vi "paint.vi"() -> ()   [LabVIEW 2017]
uses:
  <vilib>/Utility/inputDevices.llb/mouseAcquire.vi
panel:
  out "Speed":i64
  in  "Speed":T1(radio)
  out "Stop Indicator":bool
  out "Reset Frame":bool
  in  "Stop":bool
  in  "Load 4":bool
  in  "Delete Image 4":bool
  in  "Load 3":bool
  in  "Delete Image 3":bool
  in  "Load 2":bool
  in  "Delete Image 2":bool
  in  "Load 1":bool
  in  "Delete Image 1":bool
  in  "Clear":bool
  out "Saved Images":T2(array[cluster])
  in  "Save":bool
  in  "Delete Line":bool
  in  "Lines":i32(listbox)
  out "Current Image":cluster{"X":i32, "Y":i32}[][](array[cluster])
  out "2D Picture":picture
  # "Click and drag the left mouse button\ninside the black box to draw."
  # "Click on a line in\nthe list to select it.\nUse the Delete Line\nbutton to delete it.\nDeleting with no\nselection clears the\nfirst line in the list."
  # "Click the Save Image and\nClear Image buttons to save or\nclear the current image"
  # "Click STOP to stop the program"
  # "Click the Load Image or Delete Image\nbuttons below one of the saved images\nto load/delete it. Use the scrollbar to\nscroll through saved images."
  # "Laser Speed"
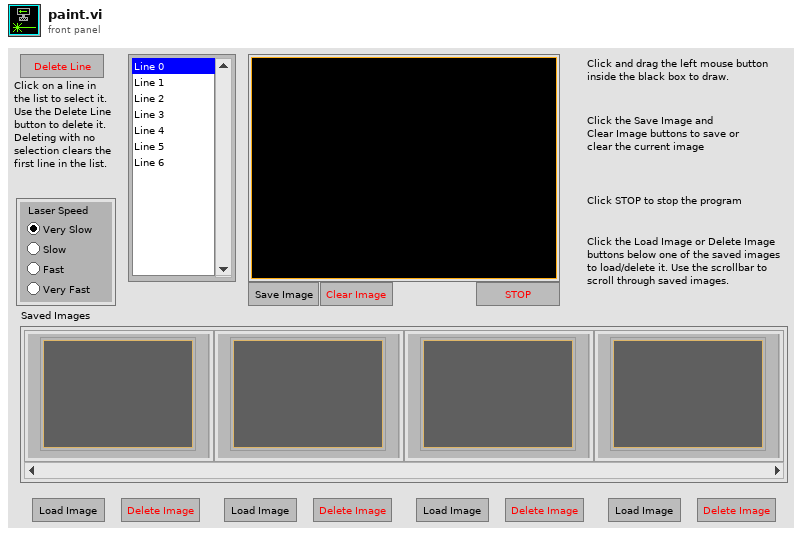
[diagram p1: front panel]
types:
  T1 = enum32{"Radio Selection 1", "Radio Selection 2", "Radio Selection 3", "Radio Selection 4"}
  T2 = cluster{"Image":picture, "Image Data":cluster{"X":dbl, "Y":dbl}[][]}[]
  T3 = enum16{"open", "replace", "create", "open or create", "replace or create", "replace or create with confirmation"}
  T4 = enum16{"big-endian, network order", "native, host order", "little-endian"}
  T5 = cluster{"Picture":picture, cluster{dbl, dbl}[][]}
  T6 = cluster{"empty picture":picture, "Array":cluster{"X":i32, "Y":i32}[][]}
  T7 = cluster{"empty picture":picture, "Array":cluster{"X":i32, "Y":i32}[][]}[]
  T8 = cluster{"button 1":bool, "button 2":bool, "button 3":bool, "button 4":bool}
  T9 = cluster{"Picture":picture, "Data Out":cluster{"X":dbl, "Y":dbl}[][]}
  T10 = cluster{"Picture":picture, "Data Out":cluster{"X":dbl, "Y":dbl}[][]}[]
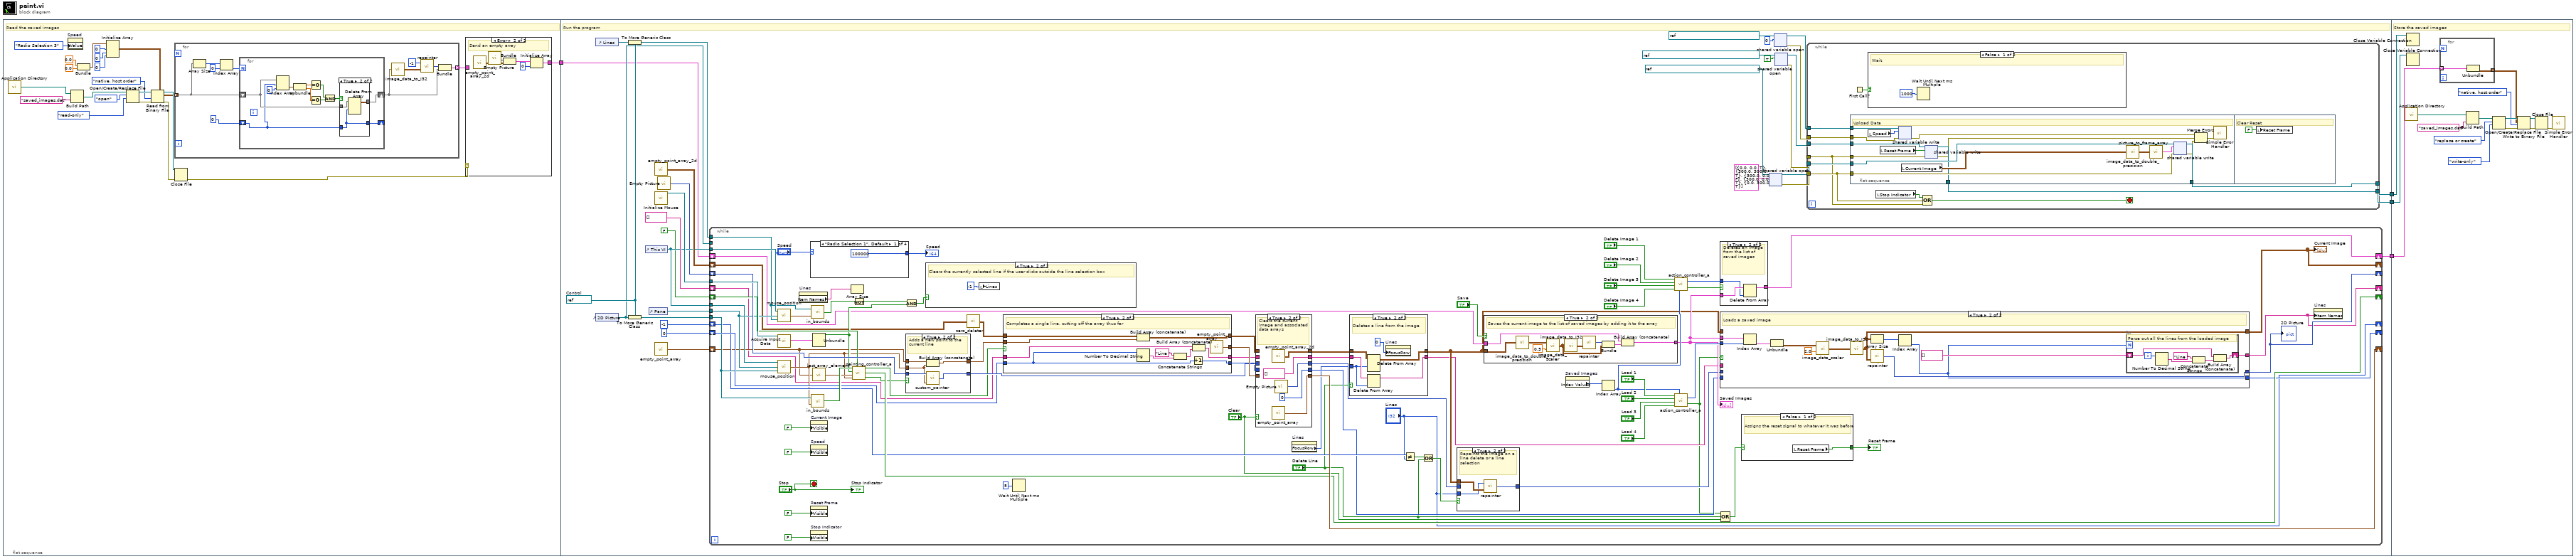
[diagram p0: block diagram]
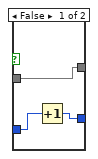
[diagram p3: hidden frame]
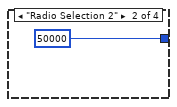
[diagram p5: hidden frame]
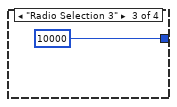
[diagram p6: hidden frame]
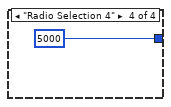
[diagram p7: hidden frame]
diagram:
  n1 = flat-sequence {
    tunnel: [w7] -> w1
    tunnel: [w69] -> w4
    tunnel: [w68] -> w3
    tunnel: [w67] -> w2
    tunnel: w1 -> [w64]
    tunnel: w4 -> [w288]
    tunnel: w3 -> [w298]
    tunnel: w2 -> [w297]
    frame #0 {
      # "Read the saved images"
      n2 = call <vilib>:"Application Directory.vi"() -> ("Application Directory"=w25:path)
      n3 = property on="Speed" class="RadioBtnsControl (strict)"("Value"=T1."Radio Selection 3" ("Speed")) -> ()  [unwired: 2 in, 2 out]
      n4 = Build Path(base path=w25, name or relative path="saved_images.dat") -> (appended path=w23:path)
      n5 = Bundle(0.0, 0.0) -> (w13:cluster{dbl, dbl})  [unwired: 1 in]
      n6 = Initialize Array(w13, 0 ("dimension size"), 0 ("dimension size"), 0 ("dimension size")) -> (w10:cluster{dbl, dbl}[][][])
      n7 = Open/Create/Replace File(file path (use dialog)=w23, operation (0:open)=T3."open", access (0:read/write)=enum16{"read/write", "read-only", "write-only"}."read-only") -> (refnum out=w22:refnum<file>, error out=w21:errorcluster)  [unwired: 3 in, 1 out]
      n8 = Read from Binary File(5:w10, 8:w21, 9:T4."native, host order" ("byte order (0:big-endian, network order)"), 11:w22) -> (0:w18:errorcluster, 2:w9:cluster{dbl, dbl}[][][], 3:w24:refnum<file>)  [unwired: 2 in, 1 out]
      n9 = for {
        tunnel: w9 -> [w37] mode=indexing
        tunnel: [w40] -> w6 mode=indexing
        n10 = Array Size(array=w37) -> (size(s)=w36:i32[])
        n11 = Index Array(array=w36, index=0) -> (element=w34:i32)
        n12 = for {
          N: w34 -> [_]
          shift-right: [w46] -> w38
          shift-left: w37 -> [w47]
          shift-right: [w44] -> _
          shift-left: 0 -> [w43]
          n13 = Index Array(array=w47, index (row)=w43, index (col)=0 ("disabled index (col)")) -> (element=w48:cluster{dbl, dbl})
          n14 = Unbundle(w48) -> (w52:dbl, w53:dbl)
          n15 = Equal To 0?(x=w52) -> (x = 0?=w50:bool)
          n16 = Equal To 0?(x=w53) -> (x = 0?=w51:bool)
          n17 = And(x=w50, y=w51) -> (x .and. y?=w45:bool)
          n18 = case shown="True" w45 {
            tunnel: w47 -> [w56 w59]
            tunnel: [w56 w58] -> w46
            tunnel: w43 -> [w54 w57]
            tunnel: [w55 w57] -> w44
            frame False {
              n19 = Increment(x=w54) -> (x+1=w55:i32)
            }
            frame True {
              n20 = Delete From Array(array=w59, index (row)=w57) -> (array with subset deleted=w58:cluster{dbl, dbl}[][])  [unwired: 2 in, 1 out]
            }
          }
        }
        n21 = call "image_data_to_I32.vi"("Data In"=w38) -> ("Data Out"=w39:cluster{"X":i32, "Y":i32}[][])
        n22 = call "repainter.vi"("Array"=w39, "Selected Line"=-1) -> ("Picture"=w41:picture)
        n23 = Bundle("Picture"=w41, w38) -> (w40:T5)  [unwired: 1 in]
      }
      n24 = Close File(refnum=w24, error in=w18) -> (error out=w8:errorcluster)  [unwired: 1 out]
      n25 = case shown="Error" w8 {
        tunnel: [w27 w28] -> w7
        tunnel: w6 -> [w27 _]
        frame No Error {
          # "Pass the data from the file on"
        }
        frame Error {
          # "Send an empty array"
          n26 = call "empty_point_array_2d.vi"() -> ("Array"=w32:cluster{"X":i32, "Y":i32}[][])
          n27 = call "Empty Picture"() -> ("empty picture"=w31:picture)
          n28 = Bundle("empty picture"=w31, "Array"=w32) -> (w30:T6)  [unwired: 1 in]
          n29 = Initialize Array(w30, 0 ("dimension size")) -> (w28:T7)
        }
      }
    }
    frame #1 {
      w81 = refnum<vi> refnum  # Control
      # "Run the program"
      n30 = control-ref of="Lines"() -> (w83:refnum<vi>)
      n31 = control-ref of="2D Picture"() -> (w78:refnum<vi>)
      n32 = To More Generic Class(target class=w81, reference=w83) -> (generic class reference=w82:refnum<vi>)
      n33 = To More Generic Class(target class=w81, reference=w78) -> (generic class reference=w80:refnum<vi>)
      n34 = control-ref of="This VI"() -> (w84:refnum<vi>)
      n35 = control-ref of="Pane"() -> (w89:refnum<vi>)
      n36 = call "empty_point_array_2d.vi"() -> ("Array"=w87:cluster{"X":i32, "Y":i32}[][])
      n37 = call <vilib>:"Initialize Mouse.vi"() -> ("device ID"=w90:refnum<k1>)  [unwired: 10 in, 1 out]
      n38 = call "empty_point_array.vi"() -> ("Array"=w88:cluster{"X":i32, "Y":i32}[])
      n39 = call "Empty Picture"() -> ("empty picture"=w79:picture)
      n40 = while {
        shift-right: [w194] -> _
        shift-left: w88 -> [w132]
        tunnel: w90 -> [w198]
        tunnel: w80 -> [w173]
        tunnel: w84 -> [w196]
        tunnel: w89 -> [w179]
        tunnel: w78 -> [_]
        shift-right: [w145] -> _
        shift-left: w79 -> [w190]
        shift-right: [w188] -> _
        shift-left: FALSE -> [w187]
        shift-right: [w139] -> _
        shift-left: w87 -> [w168]
        shift-right: [w144] -> _
        shift-left: string[] [] -> [w131]
        shift-right: [w140] -> _
        shift-left: 0 -> [w181]
        tunnel: w84 -> [w180]
        tunnel: w82 -> [w172]
        shift-right: ["Lines"] -> _
        shift-left: -1 -> [w171]
        shift-right: [w162] -> w69
        shift-left: w64 -> [w163]
        stop <- "Stop" stop-if-true
        n41 = call "mouse_position.vi"("Object"=w172, "Pane"=w179, "VI"=w180) -> ("Mouse position relative to object"=w174:cluster{"X":i32, "Y":i32})
        n42 = call-poly <vilib>:"Acquire Input Data.vi"("device ID"=w198) -> ("button info"=w197:T8)  [unwired: 15 in, 3 out]
        n43 = call "mouse_position.vi"("Object"=w173, "Pane"=w179, "VI"=w196) -> ("Mouse position relative to object"=w133:cluster{"X":i32, "Y":i32})
        n44 = property on="Lines" class="LstBox (strict)"() -> ("Item Names"=w130:string[])  [unwired: 2 in, 2 out]
        n45 = case shown="\"Radio Selection 1\", Default" "Speed" {
          tunnel: [i64 100000 i64 50000 i64 10000 i64 5000] -> w122
          frame "Radio Selection 1", Default {
          }
          frame "Radio Selection 2" {
          }
          frame "Radio Selection 3" {
          }
          frame "Radio Selection 4" {
          }
        }
        "Speed" <- w122
        n46 = property on="Current Image" class="Arr (strict)"("Visible"=FALSE) -> ()  [unwired: 2 in, 2 out]
        n47 = property on="Speed" class="DigNum (strict)"("Visible"=FALSE) -> ()  [unwired: 2 in, 2 out]
        n48 = property on="Reset Frame" class="Bool (strict)"("Visible"=FALSE) -> ()  [unwired: 2 in, 2 out]
        n49 = property on="Stop Indicator" class="Bool (strict)"("Visible"=FALSE) -> ()  [unwired: 2 in, 2 out]
        n50 = call "in_bounds.vi"("Point"=w174, "Ctl Refnum"=w172) -> ("In bounds"=w175:bool)
        n51 = call "in_bounds.vi"("Point"=w133, "Ctl Refnum"=w173) -> ("In bounds"=w185:bool)
        n52 = Unbundle(w197) -> ("button 1"=w177:bool)  [unwired: 3 out]
        n53 = call "last_array_element.vi"("Array"=w132) -> ("Last Element"=w184:cluster{"X":i32, "Y":i32})
        n54 = Array Size(array=w130) -> ()  [unwired: 1 out]
        n55 = call "painting_controller_a.vi"("In Bounds"=w185, "Mouse Clicked"=w177, "Old Point"=w184, "New Point"=w133, "Was Painting"=w187) -> ("Split"=w189:bool, "Painting"=w188:bool, "Add Point"=w186:bool)
        n56 = Not(x=w175) -> (.not. x?=w176:bool)
        n57 = And(x=w176, y=w177) -> (x .and. y?=w178:bool)
        n58 = case shown="True" w186 {
          tunnel: [w281 w283] -> w195
          tunnel: w132 -> [w281 w282]
          tunnel: [w280 w285] -> w192
          tunnel: w190 -> [w280 w286]
          tunnel: w133 -> [_ w284]
          frame False {
            # "Does not add a new point to the current line"
          }
          frame True {
            # "Adds a new point to the current line"
            n59 = Build Array (concatenate)(w282, w284) -> (w283:cluster{"X":i32, "Y":i32}[])
            n60 = call "custom_painter.vi"("Point"=w284, "Picture in"=w286) -> ("Picture out"=w285:picture)  [unwired: 1 in]
          }
        }
        n61 = case shown="True" w178 {
          frame False {
          }
          frame True {
            # "Clears the currently selected line if the user clicks outside the line selection box"
            n62 = local write "Lines"(-1 ("Lines")) -> ()
          }
        }
        n63 = call "zero_deleter.vi"("Array In"=w168) -> ("Array Out"=w167:cluster{"X":i32, "Y":i32}[][])
        n64 = case shown="True" w189 {
          tunnel: [w258 w267] -> w191
          tunnel: w167 -> [w258 w266]
          tunnel: [w257 w269] -> w193
          tunnel: w195 -> [w257 w265]
          tunnel: [w256 w263] -> w183
          tunnel: w131 -> [w256 w264]
          tunnel: [w255 w268] -> w142
          tunnel: w181 -> [w255 w262]
          frame False {
            # "Keeps the current line going"
          }
          frame True {
            # "Completes a single line, cutting off the array thus far"
            n65 = Build Array (concatenate)(w266, w265) -> (w267:cluster{"X":i32, "Y":i32}[][])
            n66 = Number To Decimal String(number=w262) -> (decimal integer string=w259:string)  [unwired: 1 in]
            n67 = Concatenate Strings("Line ", w259) -> (w260:string)
            n68 = Increment(x=w262) -> (x+1=w268:i32)
            n69 = Build Array (concatenate)(w264, w260) -> (w263:string[])
            n70 = call "empty_point_array.vi"() -> ("Array"=w269:cluster{"X":i32, "Y":i32}[])
          }
        }
        n71 = Wait Until Next ms Multiple(millisecond multiple=u32 5) -> ()  [unwired: 1 out]
        n72 = case shown="True" "Clear" {
          tunnel: [w273 w279] -> w166
          tunnel: [w274 w278] -> w194
          tunnel: w193 -> [w274 _]
          tunnel: w192 -> [w273 _]
          tunnel: [w272 w277] -> w165
          tunnel: w191 -> [w272 _]
          tunnel: [w271 string[] []] -> w182
          tunnel: w183 -> [w271 _]
          tunnel: [w270 0] -> w141
          tunnel: w142 -> [w270 _]
          frame False {
            # "Keeps the current image going"
          }
          frame True {
            # "Clears the current image and associated data arrays"
            n73 = call "empty_point_array_2d.vi"() -> ("Array"=w277:cluster{"X":i32, "Y":i32}[][])
            n74 = call "empty_point_array.vi"() -> ("Array"=w278:cluster{"X":i32, "Y":i32}[])
            n75 = call "Empty Picture"() -> ("empty picture"=w279:picture)
          }
        }
        n76 = property on="Lines" class="LstBox (strict)"() -> ("FocusRow"=w127:i32)  [unwired: 2 in, 2 out]
        n77 = case shown="True" "Delete Line" {
          tunnel: [w248 w254] -> w147
          tunnel: w165 -> [w248 w253]
          tunnel: [w247 w252] -> w143
          tunnel: w182 -> [w247 w251]
          tunnel: w127 -> [_ w250]
          frame False {
            # "Keeps the image the same"
          }
          frame True {
            # "Deletes a line from the image"
            n78 = Delete From Array(array=w253, index (row)=w250) -> (array with subset deleted=w254:cluster{"X":i32, "Y":i32}[][])  [unwired: 2 in, 1 out]
            n79 = Delete From Array(array=w251, index=w250) -> (array with subset deleted=w252:string[])  [unwired: 1 in, 1 out]
            n80 = property on="Lines" class="LstBox (strict)"("FocusRow"=0 ("Focus Row")) -> ()  [unwired: 2 in, 2 out]
          }
        }
        n81 = Not Equal?(x=w171, y="Lines") -> (x != y?=w170:bool)
        n82 = Or(x=w170, y="Delete Line") -> (x .or. y?=w169:bool)
        n83 = case shown="True" w169 {
          tunnel: w166 -> [w243 _]
          tunnel: [w243 w246] -> w146
          tunnel: w147 -> [_ w245]
          tunnel: "Lines" -> [_ w244]
          frame False {
            # "Does not repaint the image"
          }
          frame True {
            # "Repaints the image on a line delete or a line selection"
            n84 = call "repainter.vi"("Array"=w245, "Selected Line"=w244) -> ("Picture"=w246:picture)
          }
        }
        n85 = case shown="True" "Save" {
          tunnel: [w232 w240] -> w148
          tunnel: w163 -> [w232 w241]
          tunnel: w147 -> [_ w235]
          frame False {
            # "Leaves the list of saved images alone"
          }
          frame True {
            # "Saves the current image to the list of saved images by adding it to the array"
            n86 = call "image_data_to_double_precision.vi"("Data In"=w235) -> ("Data Out"=w234:cluster{"X":dbl, "Y":dbl}[][])
            n87 = call "image_data_scaler.vi"("Scale"=0.5, "Data In"=w234) -> ("Data Out"=w237:cluster{"X":dbl, "Y":dbl}[][])
            n88 = call "image_data_to_I32.vi"("Data In"=w237) -> ("Data Out"=w236:cluster{"X":i32, "Y":i32}[][])
            n89 = call "repainter.vi"("Array"=w236) -> ("Picture"=w238:picture)  [unwired: 1 in]
            n90 = Bundle("Picture"=w238, "Data Out"=w237) -> (w233:T9)  [unwired: 1 in]
            n91 = Build Array (concatenate)(w241, w233) -> (w240:T10)
          }
        }
        "Saved Images" <- w148
        n92 = property on="Saved Images" class="Arr (strict)"() -> ("Index Values"=w161:u32[])  [unwired: 2 in, 2 out]
        n93 = Index Array(array=w161) -> (element=w150:u32)  [unwired: 1 in]
        n94 = call "action_controller_a.vi"("Action 1"="Delete Image 1", "Action 2"="Delete Image 2", "Action 3"="Delete Image 3", "Action 4"="Delete Image 4", "First Visible Index"=w150) -> ("Index"=w158:i32, "Action"=w157:bool)
        n95 = call "action_controller_a.vi"("Action 1"="Load 1", "Action 2"="Load 2", "Action 3"="Load 3", "Action 4"="Load 4", "First Visible Index"=w150) -> ("Index"=w149:i32, "Action"=w138:bool)
        n96 = case shown="True" w157 {
          tunnel: [w228 w230] -> w162
          tunnel: w148 -> [w228 w231]
          tunnel: w158 -> [_ w229]
          frame False {
            # "Does not delete anything"
          }
          frame True {
            # "Deletes an image from the list of saved images"
            n97 = Delete From Array(array=w231, index=w229) -> (array with subset deleted=w230:T10)  [unwired: 1 in, 1 out]
          }
        }
        n98 = case shown="True" w138 {
          tunnel: w149 -> [_ w221]
          tunnel: w148 -> [_ w220]
          tunnel: [w209 w214] -> w139
          tunnel: w147 -> [w209 _]
          tunnel: [w208 w218] -> w145
          tunnel: w146 -> [w208 _]
          tunnel: [w207 w212] -> w144
          tunnel: w143 -> [w207 _]
          tunnel: w141 -> [w206 _]
          tunnel: [w206 w210] -> w140
          frame False {
            # "Does not load anything"
          }
          frame True {
            # "Loads a saved image"
            n99 = Index Array(array=w220, index=w221) -> (element=w219:T9)
            n100 = Unbundle(w219) -> ("Data Out"=w216:cluster{"X":dbl, "Y":dbl}[][])  [unwired: 1 out]
            n101 = call "image_data_scaler.vi"("Scale"=2.0, "Data In"=w216) -> ("Data Out"=w215:cluster{"X":dbl, "Y":dbl}[][])
            n102 = call "image_data_to_I32.vi"("Data In"=w215) -> ("Data Out"=w214:cluster{"X":i32, "Y":i32}[][])
            n103 = Array Size(array=w214) -> (size(s)=w213:i32[])
            n104 = call "repainter.vi"("Array"=w214) -> ("Picture"=w218:picture)  [unwired: 1 in]
            n105 = Index Array(array=w213) -> (element=w210:i32)  [unwired: 1 in]
            n106 = for {
              N: w210 -> [_]
              shift-right: [w222] -> w212
              shift-left: string[] [] -> [w223]
              i -> [w227]
              # "Parse out all the lines from the loaded image"
              n107 = Number To Decimal String(number=w227) -> (decimal integer string=w225:string)  [unwired: 1 in]
              n108 = Concatenate Strings("Line ", w225) -> (w224:string)
              n109 = Build Array (concatenate)(w223, w224) -> (w222:string[])
            }
          }
        }
        "2D Picture" <- w145
        "Current Image" <- w139
        n110 = Compound Arithmetic op=OR(w138, "Delete Line", "Clear") -> (w135:bool)
        n111 = case shown="False" w135 {
          selector: w135 -> [_ w205]
          tunnel: [w204 w205] -> w134
          frame False {
            # "Assigns the reset signal to whatever it was before"
            n112 = local read "Reset Frame"() -> (w204:bool)
          }
          frame True {
            # "Tells the myRIO to reset the image data on image load, line delete, or image clear"
          }
        }
        "Reset Frame" <- w134
        n113 = property on="Lines" class="LstBox (strict)"("Item Names"=w144) -> ()  [unwired: 2 in, 2 out]
        "Stop Indicator" <- "Stop"
      }
      n114 = shared-variable-open(refnum<k21> "ni.var.psp://reflectech/FrameArray/FrameArray" ("shared variable refnum in"), cluster{"\nX":dbl, " Y":dbl, "On/Off":bool}[] [{"\nX"=0.0, " Y"=0.0, "On/Off"=TRUE}, {"\nX"=300.0, " Y"=300.0, "On/Off"=TRUE}, {"\nX"=300.0, " Y"=0.0, "On/Off"=FALSE}, {"\nX"=300.0, " Y"=0.0, "On/Off"=TRUE}, {"\nX"=0.0, " Y"=300.0, "On/Off"=TRUE}] ("Array 2")) -> (w75:refnum<k21>, w66:errorcluster)  [unwired: 2 in]
      n115 = shared-variable-open(refnum<k21> "ni.var.psp://reflectech/Speed/Speed" ("shared variable refnum in"), i64 0 ("Numeric")) -> (w61:refnum<k21>, w60:errorcluster)  [unwired: 2 in]
      n116 = shared-variable-open(refnum<k21> "ni.var.psp://reflectech/Reset Frame/Reset Frame" ("shared variable refnum in"), TRUE) -> (w72:refnum<k21>, w65:errorcluster)  [unwired: 2 in]
      n117 = while {
        tunnel: w75 -> [w101]
        tunnel: w66 -> [w97]
        tunnel: w72 -> [w100]
        tunnel: w65 -> [w96]
        tunnel: [w94] -> w68
        tunnel: [w93] -> w67
        tunnel: w61 -> [w92]
        tunnel: w60 -> [w91]
        stop <- w95 stop-if-true
        n118 = flat-sequence {
          tunnel: w101 -> [w119]
          tunnel: w97 -> [w118]
          tunnel: w100 -> [w117]
          tunnel: w96 -> [w116]
          tunnel: [w111] -> w94
          tunnel: [w110] -> w93
          tunnel: w92 -> [w108]
          tunnel: w91 -> [w107]
          frame #0 {
            # "Upload Data"
            n119 = local read "Speed"() -> (w109:i64)
            n120 = local read "Reset Frame"() -> (w114:bool)
            n121 = shared-variable-write(w108, w107, w109) -> (w106:errorcluster)  [unwired: 1 out]
            n122 = local read "Current Image"() -> (w113:cluster{"X":i32, "Y":i32}[][])
            n123 = shared-variable-write(w117, w116, w114) -> (w111:refnum<k21>, w104:errorcluster)
            n124 = call "image_data_to_double_precision.vi"("Data In"=w113) -> ("Data Out"=w112:cluster{"X":dbl, "Y":dbl}[][])
            n125 = call "picture_to_frame_array.vi"("Image In"=w112) -> ("Image Out"=w115:cluster{"X":dbl, "Y":dbl, "Laser":bool}[])
            n126 = shared-variable-write(w119, w118, w115) -> (w110:refnum<k21>, w105:errorcluster)
            n127 = Merge Errors(w106, w104, w105) -> (w103:errorcluster)
            n128 = call <vilib>:"Simple Error Handler.vi"("error in (no error)"=w103) -> ()  [unwired: 4 in, 5 out]
          }
          frame #1 {
            # "Clear Reset"
            n129 = local write "Reset Frame"(FALSE ("Reset Frame")) -> ()
          }
        }
        n130 = First Call?() -> (First Call?: T/F=w99:bool)
        n131 = case shown="False" w99 {
          frame False {
            # "Wait"
            n132 = Wait Until Next ms Multiple(millisecond multiple=u32 1000) -> ()  [unwired: 1 out]
          }
          frame True {
            # "Don't wait on the first time so that if the shared variables are not opened correclty, this loop stops running"
          }
        }
        n133 = local read "Stop Indicator"() -> (w98:bool)
        n134 = Compound Arithmetic op=OR(w98, w97, w96) -> (w95:bool)
      }
    }
    frame #2 {
      # "Store the saved images"
      n135 = call <vilib>:"Application Directory.vi"() -> ("Application Directory"=w295:path)
      n136 = Close Variable Connection(11:w297) -> ()  [unwired: 1 in, 1 out]
      n137 = Close Variable Connection(11:w298) -> ()  [unwired: 1 in, 1 out]
      n138 = for {
        tunnel: w288 -> [w303] mode=indexing
        tunnel: [w302] -> w287 mode=indexing
        n139 = Unbundle(w303) -> ("Array"=w302:cluster{"X":dbl, "Y":dbl}[][])  [unwired: 1 out]
      }
      n140 = Build Path(base path=w295, name or relative path="saved_images.dat") -> (appended path=w294:path)
      n141 = Open/Create/Replace File(file path (use dialog)=w294, operation (0:open)=T3."replace or create", access (0:read/write)=enum16{"read/write", "read-only", "write-only"}."write-only") -> (refnum out=w291:refnum<file>, error out=w290:errorcluster)  [unwired: 3 in, 1 out]
      n142 = Write to Binary File(file (use dialog)=w291, data=w287, error in=w290, 9:T4."native, host order" ("byte order (0:big-endian, network order)")) -> (refnum out=w299:refnum<file>, error out=w300:errorcluster)  [unwired: 2 in, 1 out]
      n143 = Close File(refnum=w299, error in=w300) -> (error out=w301:errorcluster)  [unwired: 1 out]
      n144 = call <vilib>:"Simple Error Handler.vi"("error in (no error)"=w301) -> ()  [unwired: 4 in, 5 out]
    }
  }
